vi "Set Tag.vi"(8 "error in":errorcluster, 10 "Tag":variant, 11 "Cell in":refnum<class "Cell.lvclass">) -> (0 "error out":errorcluster, 3 "Cell out":refnum<class "Cell.lvclass">)   [LabVIEW 2024, in "SourceGrid.lvlib" / "Cell.lvclass"]
uses:
  Cell.lvclass
  Cell.lvclass/Cell.ctl
  D:/git/Sourcegrid-LabVIEW/dll/SourceGrid.dll
  dll/SourceGrid.dll
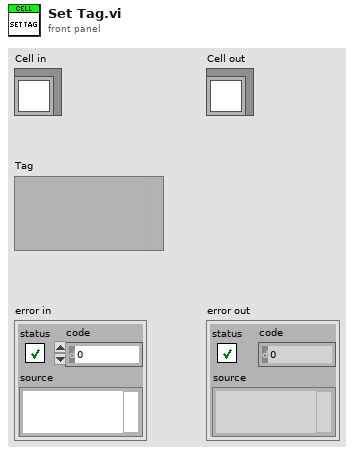
[diagram p1: front panel]
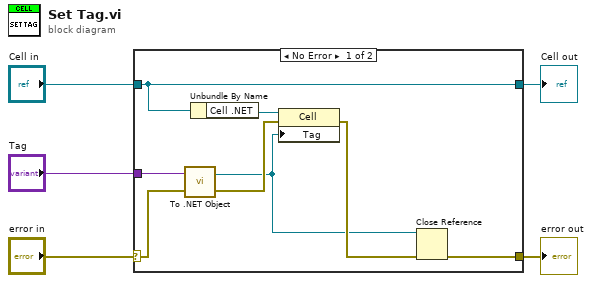
[diagram p0: block diagram]
diagram:
  n1 = case shown="No Error" "error in" {
    selector: "error in" -> [w12 w14]
    tunnel: [w7 w14] -> w4
    tunnel: [w11 w15] -> w2
    tunnel: "Cell in" -> [w11 w15]
    tunnel: "Tag" -> [w13 _]
    frame No Error {
      n2 = call <vilib>:"To .NET Object.vi"("error in (no error)"=w12, "anything"=w13) -> ("error out"=w10:errorcluster, ".NET object"=w6:refnum<k24>)
      n3 = Unbundle By Name(w11) -> ("Cell .NET"=w9:refnum<k24>)
      n4 = property class="Cell"(reference=w9, error in=w10, "Tag"=w6) -> (error out=w8:errorcluster)  [unwired: 1 out]
      n5 = Close Reference(reference=w6, error in (no error)=w8) -> (error out=w7:errorcluster)
    }
    frame Error {
    }
  }
  "error out" <- w4
  "Cell out" <- w2
